vi "Update Log.vi"(8 "error in (no error)":errorcluster, 10 "Lab notebook entry":string, 11 "Log Record in":refnum<class "Log Record.lvclass">) -> (0 "error out":errorcluster, 2 "path":path, 3 "Log Record out":refnum<class "Log Record.lvclass">)   [LabVIEW 2024, in "Log Record.lvclass"]
uses:
  Log Record.lvclass
  C:/GitHub/LabActor/Worker/Worker Actor/Worker Actor.lvclass
  Worker/Worker Actor/Worker Actor.lvclass/Worker Actor.ctl
  Worker/Worker Actor/Read Project folder .vi
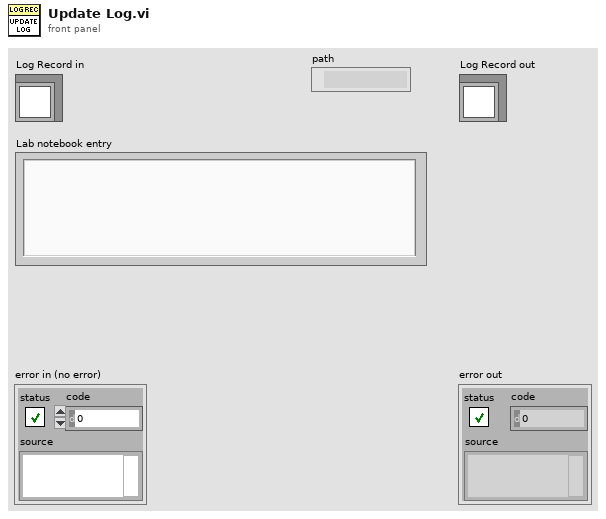
[diagram p1: front panel]
types:
  T1 = enum16{"open", "replace", "create", "open or create", "replace or create", "replace or create with confirmation"}
  T2 = typedef "Experiment info.ctl" = cluster{"attendee":string[], "title":string, "magnet_System":string, "proposal_Number":string, "proposal_Title":string, "facility":string, "pi":string, "dtstart":string, "dtend":string, "dtstamp":string, "location":string, "summary":string, "pid":string, "support":string, "uid":string, "start":u64, "id":u64}
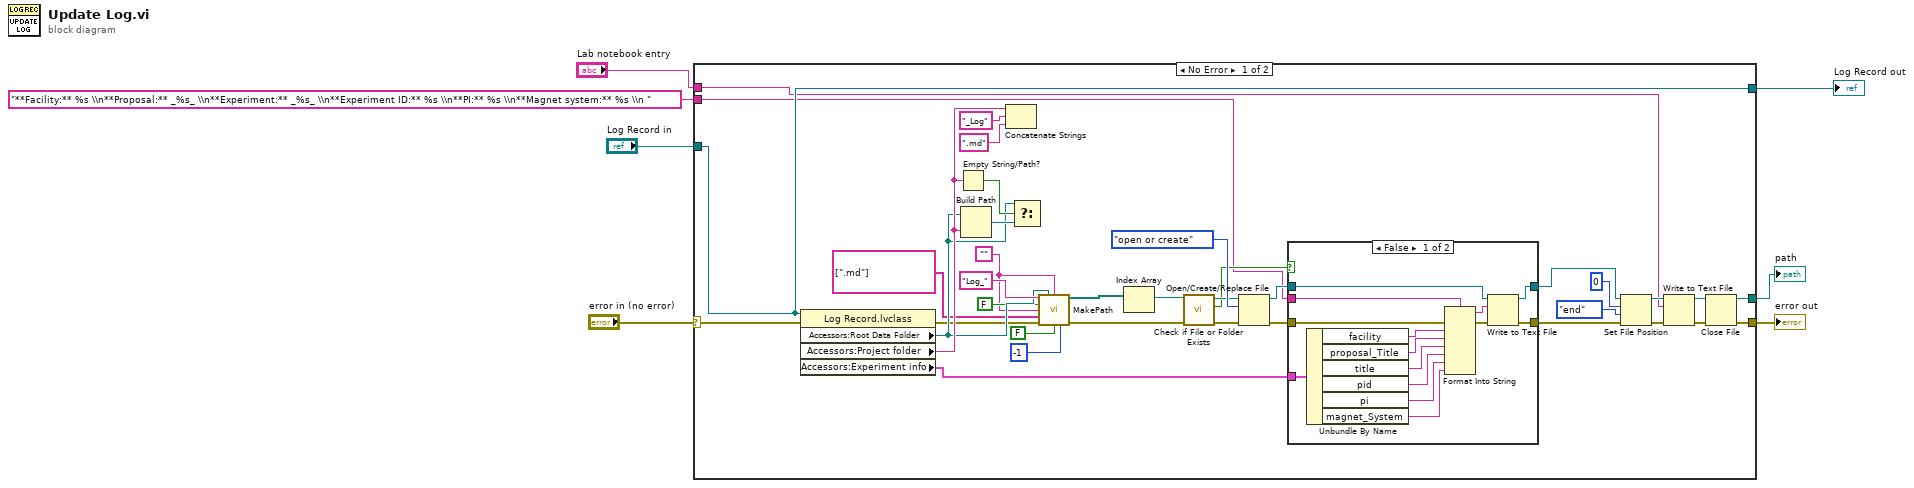
[diagram p0: block diagram]
diagram:
  n1 = case shown="No Error" "error in (no error)" {
    selector: "error in (no error)" -> [w32 w62]
    tunnel: [w31 w62] -> w6
    tunnel: [w44 w61] -> w4
    tunnel: "Log Record in" -> [w44 w61]
    tunnel: "Lab notebook entry" -> [w35 _]
    tunnel: [w30 _] -> w2
    tunnel: "**Facility:** %s \\n**Proposal:** _%s_ \\n**Experiment:** _%s_ \\n**Experiment ID:** %s \\n**PI:** %s \\n**Magnet system:** %s \\n " ("format string") -> [w19 _]
    frame No Error {
      w12 = ""
      n2 = property class="Log Record.lvclass"(reference=w44, error in=w32) -> (error out=w13:errorcluster, "Accessors:Root Data Folder"=w16:path, "Accessors:Project folder "=w29:string, "Accessors:Experiment info"=w21:T2)  [unwired: 1 out]
      n3 = Empty String/Path?(string/path=w29) -> (empty?=w42:bool)
      n4 = Build Path(base path=w16, name or relative path=w29) -> (appended path=w43:path)
      n5 = Concatenate Strings(w29, "_Log" ("string"), ".md" ("string")) -> ()  [unwired: 1 out]
      n6 = Select(t=w16, s=w42, f=w43) -> ()  [unwired: 1 out]
      n7 = call "MakePath.vi"("File Prefix"="Log_", "Root Data Folder"=w16, "Index file"=w12, "Interactive"=FALSE, "File middle"=w12, "Extentions"=string[] [".md"], "Error In"=w13, "Include time"=FALSE, "Index digits"=-1) -> ("Paths out"=w9:path[], "Error Out"=w26:errorcluster)  [unwired: 2 in, 3 out]
      n8 = Index Array(array=w9) -> (element=w8:path)  [unwired: 1 in]
      n9 = call <vilib>:"Check if File or Folder Exists.vi"("error in (no error)"=w26, "path"=w8) -> ("error out"=w25:errorcluster, "file or folder exists?"=w24:bool, "dup path"=w27:path)  [unwired: 7 in]
      n10 = Open/Create/Replace File(file path (use dialog)=w27, error in=w25, operation (0:open)=T1."open or create") -> (refnum out=w22:refnum<file>, error out=w23:errorcluster)  [unwired: 3 in, 1 out]
      n11 = case shown="False" w24 {
        tunnel: w23 -> [w51 w60]
        tunnel: w22 -> [w49 w59]
        tunnel: w21 -> [w58 _]
        tunnel: w19 -> [w57 _]
        tunnel: [w48 w60] -> w20
        tunnel: [w47 w59] -> w18
        frame False {
          n12 = Unbundle By Name(w58) -> ("facility"=w56:string, "proposal_Title"=w55:string, "title"=w54:string, "pid"=w53:string, "pi"=w45:string, "magnet_System"=w52:string)
          n13 = Format Into String(format string=w57, error in=w51, w56, w55, w54, w53, w45, w52) -> (resulting string=w46:string, error out=w50:errorcluster)  [unwired: 1 in]
          n14 = Write to Text File(file (use dialog)=w49, text=w46, error in=w50) -> (refnum out=w47:refnum<file>, error out=w48:errorcluster)  [unwired: 1 in, 1 out]
        }
        frame True {
        }
      }
      n15 = Set File Position(offset (in bytes) (0)=i64 0, refnum=w18, from (0:start)=enum16{"start", "end", "current"}."end", error in=w20) -> (refnum out=w37:refnum<file>, error out=w36:errorcluster)
      n16 = Write to Text File(file (use dialog)=w37, text=w35, error in=w36) -> (refnum out=w33:refnum<file>, error out=w34:errorcluster)  [unwired: 1 in, 1 out]
      n17 = Close File(refnum=w33, error in=w34) -> (path=w30:path, error out=w31:errorcluster)
    }
    frame Error {
    }
  }
  "error out" <- w6
  "Log Record out" <- w4
  "path" <- w2
